vi "Create.vi"(8 "error in (no error)":errorcluster, 9 "Group":refnum<class "Group.lvclass">, 10 "Parent Name":string) -> (0 "error out":errorcluster, 3 "Data Logger Module out":refnum<class "Data Logger Module.lvclass">)   [LabVIEW 2020, in "VolatusData.lvlib" / "Data Logger Module.lvclass"]
uses:
  Data Logger Module.lvclass
  Data Logger Module.lvclass/Data Logger Module.ctl
  lv-vecto/Vecto/Group/Group.lvclass
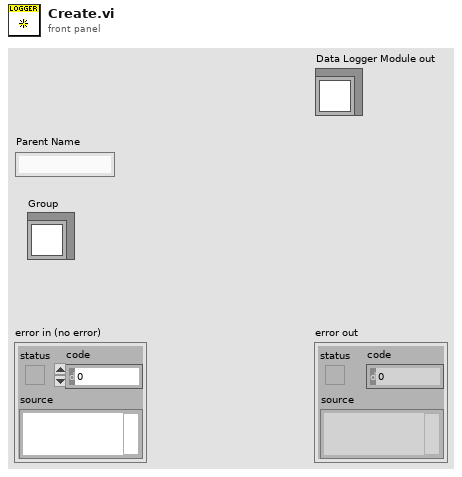
[diagram p1: front panel]
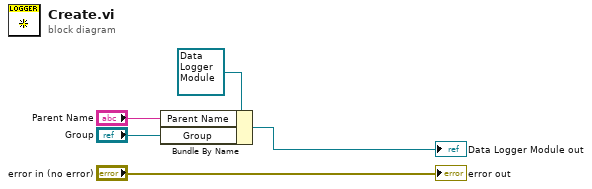
[diagram p0: block diagram]
diagram:
  n1 = Bundle By Name(cluster=refnum<class "Data Logger Module.lvclass"> refnum ("Data Logger Module in"), "Parent Name"="Parent Name", "Group"="Group") -> (→"Data Logger Module out":refnum<class "Data Logger Module.lvclass">)
  "error out" <- "error in (no error)"
